vi "get_centroid.vi"(8 "error in (no error)":errorcluster, 11 "PointCollection in":refnum<class "PointCollection.lvclass">) -> (0 "error out":errorcluster, 2 "centroid":dbl[](array[numeric]), 3 "PointCollection out":refnum<class "PointCollection.lvclass">)   [LabVIEW 2010, in "PointCollection.lvclass"]
uses:
  PointCollection.lvclass
  <vilib>/Analysis/NI_AALBase.lvlib
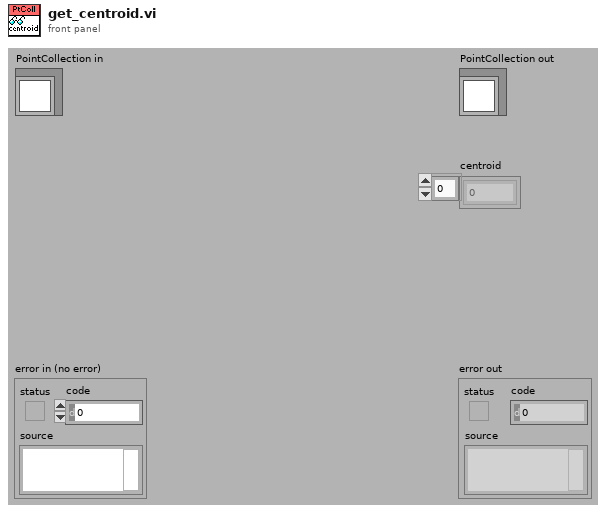
[diagram p1: front panel]
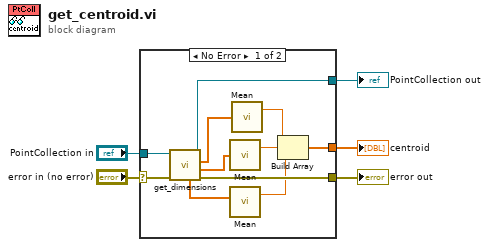
[diagram p0: block diagram]
diagram:
  n1 = case shown="No Error" "error in (no error)" {
    selector: "error in (no error)" -> [w16 w18]
    tunnel: [w15 w18] -> w4
    tunnel: [w13 w17] -> w2
    tunnel: "PointCollection in" -> [w14 w17]
    tunnel: [w6 _] -> w1
    frame No Error {
      n2 = call-dynamic "get_dimensions.vi"("error in (no error)"=w16, "PointCollection in"=w14) -> ("error out"=w15:errorcluster, "y"=w11:dbl[], "x"=w12:dbl[], "PointCollection out"=w13:refnum<class "PointCollection.lvclass">, "z"=w10:dbl[])  [unwired: 4 in, 1 out]
      n3 = call <vilib>:"Mean.vi"("X"=w11) -> ("mean"=w8:dbl)  [unwired: 1 out]
      n4 = call <vilib>:"Mean.vi"("X"=w10) -> ("mean"=w7:dbl)  [unwired: 1 out]
      n5 = call <vilib>:"Mean.vi"("X"=w12) -> ("mean"=w9:dbl)  [unwired: 1 out]
      n6 = Build Array(w9, w8, w7) -> (w6:dbl[])
    }
    frame Error {
    }
  }
  "error out" <- w4
  "PointCollection out" <- w2
  "centroid" <- w1
